vi "InsertEntuseNoTransaction.vi"() -> (10 "Entity":string)   [LabVIEW 2012]
uses:
  <vilib>/addons/database/Connection.llb/DB Tools Open Connec (Path).vi
  <vilib>/addons/database/Connection.llb/Conn Execute.vi
  <vilib>/addons/database/Recordset.llb/Rec Fetch Recordset Data (R).vi
  <vilib>/addons/database/Recordset.llb/Rec Destroy - Connection.vi
  <vilib>/addons/database/_DB Variant To Data/Database Variant To Data.xnode
  <vilib>/addons/database/NI_Database_API.lvlib
panel:
  in  "Entity":string
  out "array":string[][](array[string])
  out "error out":errorcluster
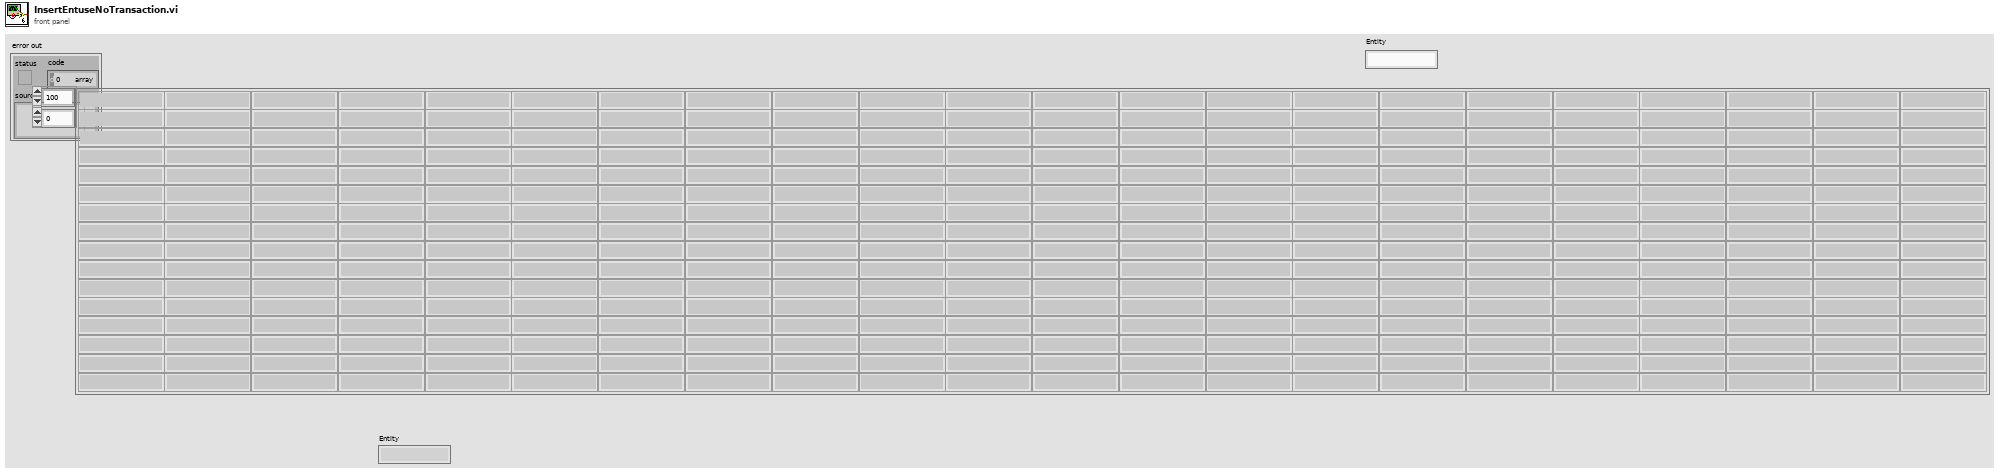
[diagram p1: front panel]
types:
  T1 = typedef "NI_Database_API.lvlib/Conn ObjectReference.ctl" = refnum<k1>
  T2 = typedef "NI_Database_API.lvlib/Rec ObjectReference.ctl" = refnum<k1>
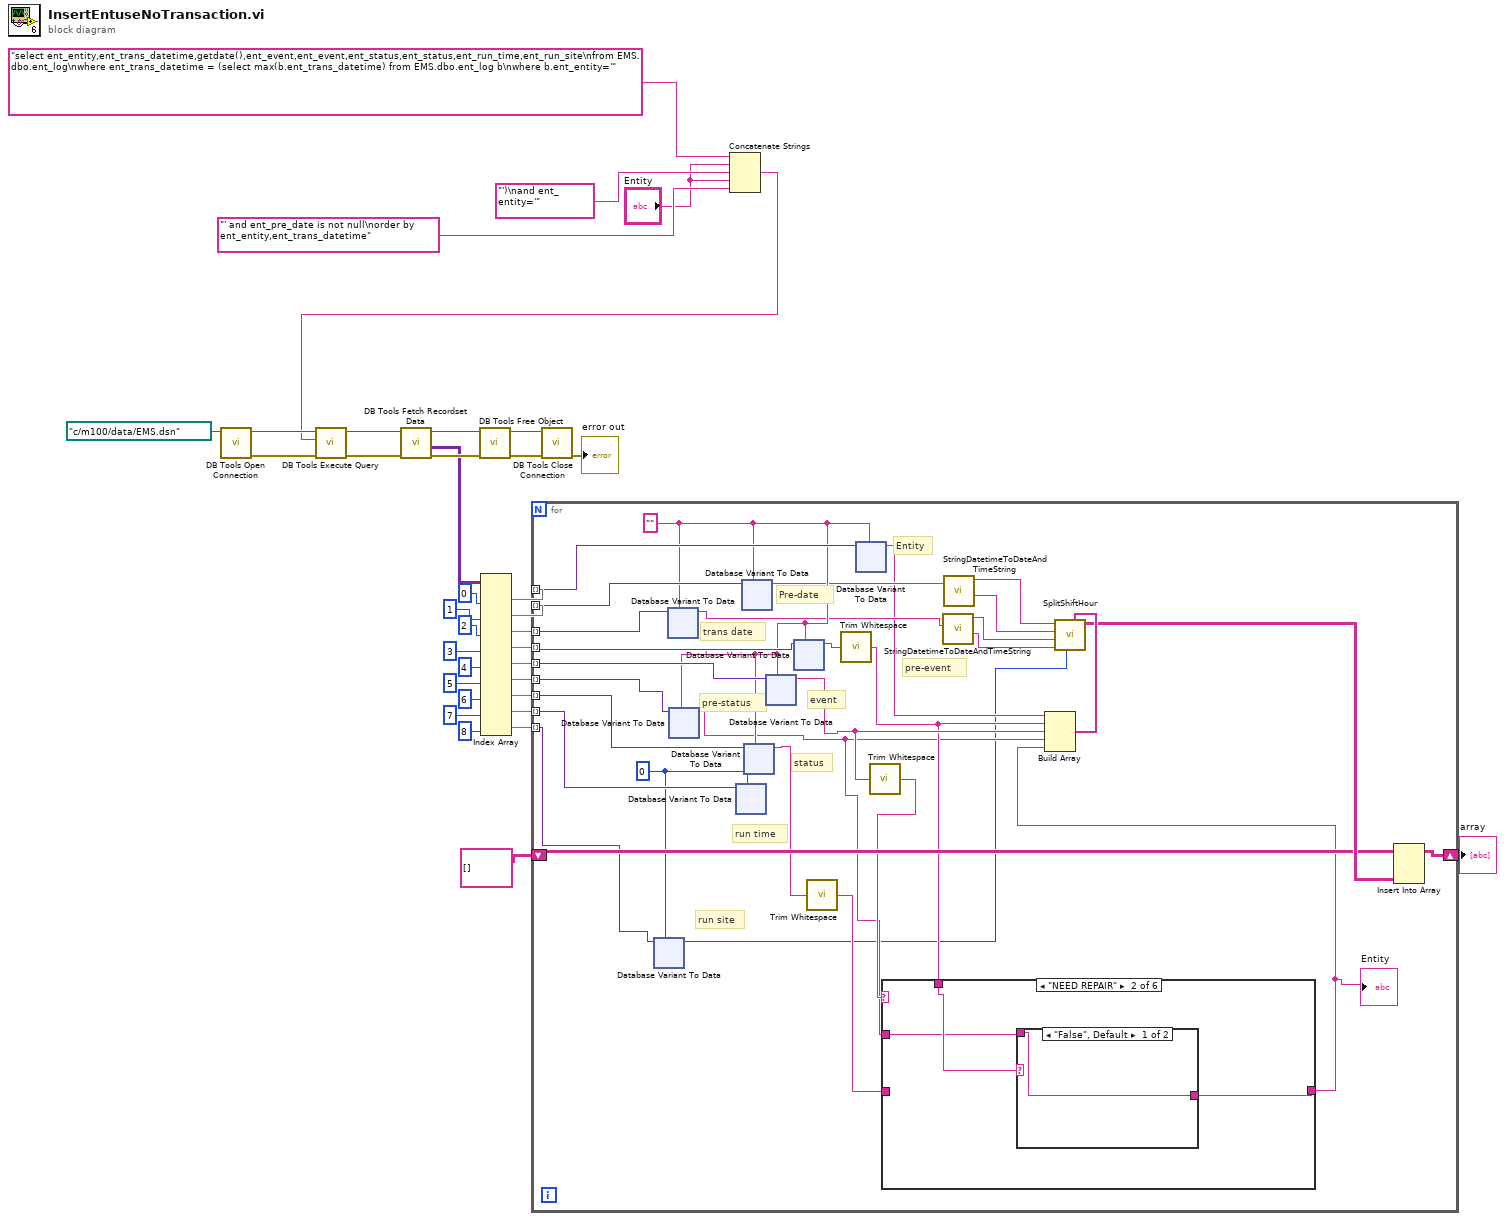
[diagram p0: block diagram]
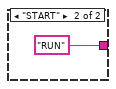
[diagram p3: hidden frame]
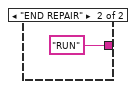
[diagram p4: hidden frame]
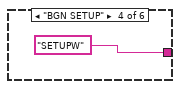
[diagram p7: hidden frame]
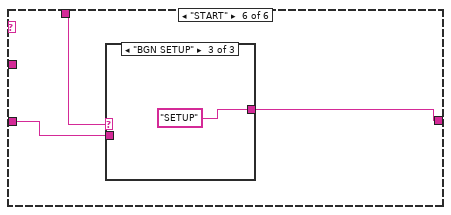
[diagram p9: hidden frame]
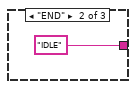
[diagram p11: hidden frame]
diagram:
  n1 = call-poly <vilib>:"DB Tools Open Connection.vi"("connection information"=path "c:/m100/data/EMS.dsn") -> ("error out"=w32:errorcluster, "connection reference"=w36:T1)  [unwired: 7 in]
  n2 = Concatenate Strings("select ent_entity,ent_trans_datetime,getdate(),ent_event,ent_event,ent_status,ent_status,ent_run_time,ent_run_site\nfrom EMS.dbo.ent_log\nwhere ent_trans_datetime = (select max(b.ent_trans_datetime) from EMS.dbo.ent_log b\nwhere b.ent_entity='" ("string"), "Entity", "')\nand ent_entity='" ("string"), "Entity", "' and ent_pre_date is not null\norder by ent_entity,ent_trans_datetime" ("string")) -> (w3:string)
  n3 = call-poly <vilib>:"DB Tools Execute Query.vi"("error in (no error)"=w32, "SQL query"=w3, "connection reference"=w36) -> ("error out"=w31:errorcluster, "recordset reference"=w35:T2)  [unwired: 5 in]
  n4 = call-poly <vilib>:"DB Tools Fetch Recordset Data.vi"("error in (no error)"=w31, "recordset reference"=w35) -> ("error out"=w30:errorcluster, "recordset data"=w26:variant[][], "recordset reference out"=w34:T2)  [unwired: 3 in]
  n5 = call-poly <vilib>:"DB Tools Free Object.vi"("error in (no error)"=w30, "recordset reference"=w34) -> ("error out"=w29:errorcluster, "connection reference"=w33:T1)  [unwired: 8 in]
  n6 = Index Array(array=w26, index (col) #1=0 ("disabled index (col)"), index (col) #2=1 ("index (col)"), index (col) #3=2 ("index (col)"), index (col) #4=3 ("index (col)"), index (col) #5=4 ("index (col)"), index (col) #6=5 ("index (col)"), index (col) #7=6 ("index (col)"), index (col) #8=7 ("index (col)"), index (col) #9=8 ("index (col)")) -> (element #1=w19:variant[], element #2=w18:variant[], element #3=w17:variant[], element #4=w16:variant[], element #5=w15:variant[], element #6=w14:variant[], element #7=w13:variant[], element #8=w10:variant[], element #9=w6:variant[])  [unwired: 9 in]
  n7 = for {
    tunnel: w19 -> [w67] mode=indexing
    tunnel: w18 -> [w66] mode=indexing
    tunnel: w17 -> [w65] mode=indexing
    tunnel: w16 -> [w64] mode=indexing
    tunnel: w15 -> [w63] mode=indexing
    tunnel: w14 -> [w62] mode=indexing
    tunnel: w13 -> [w61] mode=indexing
    tunnel: w10 -> [w52] mode=indexing
    shift-right: [w49] -> w8
    shift-left: string[][] [] ("array") -> [w48]
    tunnel: w6 -> [w40] mode=indexing
    w39 = 0
    w60 = ""
    # "run site"
    # "run time"
    # "status"
    # "pre-status"
    # "event"
    # "pre-event"
    # "trans date"
    # "Pre-date"
    # "Entity"
    n8 = xnode "Database Variant To Data"("database variant"=w40, "type"=w39) -> ("data"=w37:i32)  [unwired: 1 in, 1 out]
    n9 = xnode "Database Variant To Data"("database variant"=w65, "type"=w60) -> ("data"=w58:string)  [unwired: 1 in, 1 out]
    n10 = xnode "Database Variant To Data"("database variant"=w62, "type"=w60) -> ("data"=w41:string)  [unwired: 1 in, 1 out]
    n11 = xnode "Database Variant To Data"("database variant"=w52, "type"=w39) -> ()  [unwired: 1 in, 2 out]
    n12 = xnode "Database Variant To Data"("database variant"=w66, "type"=w60) -> ("data"=w59:string)  [unwired: 1 in, 1 out]
    n13 = xnode "Database Variant To Data"("database variant"=w61, "type"=w60) -> ("data"=w45:string)  [unwired: 1 in, 1 out]
    n14 = xnode "Database Variant To Data"("database variant"=w63, "type"=w60) -> ("data"=w47:string)  [unwired: 1 in, 1 out]
    n15 = xnode "Database Variant To Data"("database variant"=w64, "type"=w60) -> ("data"=w43:string)  [unwired: 1 in, 1 out]
    n16 = call <vilib>:"Trim Whitespace.vi"("string"=w45) -> ("trimmed string"=w44:string)  [unwired: 1 in]
    n17 = call <vilib>:"Trim Whitespace.vi"("string"=w43) -> ("trimmed string"=w42:string)  [unwired: 1 in]
    n18 = xnode "Database Variant To Data"("database variant"=w67, "type"=w60) -> ("data"=w53:string)  [unwired: 1 in, 1 out]
    n19 = call <vilib>:"Trim Whitespace.vi"("string"=w47) -> ("trimmed string"=w46:string)  [unwired: 1 in]
    n20 = case shown="\"NEED REPAIR\"" w46 {
      tunnel: [w102 w107 w112 "SETUPW" w118 w120] -> w38
      tunnel: w44 -> [w101 _ w113 _ _ w119]
      tunnel: w42 -> [w103 w108 w114 _ _ w121]
      tunnel: w41 -> [w100 w106 w111 _ w118 _]
      frame "END", Default {
        n21 = case shown="\"False\", Default" w103 {
          tunnel: [w104 "RUN"] -> w102
          tunnel: w101 -> [_ _]
          tunnel: w100 -> [w104 _]
          frame "False", Default {
          }
          frame "START" {
          }
        }
      }
      frame "NEED REPAIR" {
        n22 = case shown="\"False\", Default" w108 {
          tunnel: [w109 "RUN"] -> w107
          tunnel: w106 -> [w109 _]
          frame "False", Default {
          }
          frame "END REPAIR" {
          }
        }
      }
      frame "BGN REPAIR" {
        n23 = case shown="\"START\"" w114 {
          tunnel: w113 -> [_ _]
          tunnel: [w115 w116] -> w112
          tunnel: w111 -> [w115 w116]
          frame "False", Default {
          }
          frame "START" {
          }
        }
      }
      frame "BGN SETUP" {
      }
      frame "END REPAIR" {
      }
      frame "START" {
        n24 = case shown="\"BGN SETUP\"" w121 {
          tunnel: [w122 "IDLE" "SETUP"] -> w120
          tunnel: w119 -> [w122 _ _]
          frame "False", Default {
          }
          frame "END" {
          }
          frame "BGN SETUP" {
          }
        }
      }
    }
    "Entity" <- w38
    n25 = call "StringDatetimeToDateAndTimeString.vi"("String"=w58) -> ("Time String"=w54:string, "Date String"=w55:string)  [unwired: 8 in, 1 out]
    n26 = call "StringDatetimeToDateAndTimeString.vi"("String"=w59) -> ("Time String"=w56:string, "Date String"=w57:string)  [unwired: 8 in, 1 out]
    n27 = Build Array(w53, w42, w47, w41, w38) -> (w51:string[])
    n28 = call "SplitShiftHour.vi"("BasicData"=w51, "Site"=w37, "EndTime 2"=w54, "date string"=w55, "BegTime"=w56, "BegDate"=w57) -> ("array"=w50:string[][])  [unwired: 5 in]
    n29 = Insert Into Array(array=w48, new element=w50) -> (w49:string[][])  [unwired: 2 in]
  }
  "array" <- w8
  n30 = call <vilib>:"DB Tools Close Connection.vi"("error in (no error)"=w29, "connection reference"=w33) -> ("error out"=→"error out":errorcluster)  [unwired: 5 in]
